vi "ICM Extract Data.vi"(8 "error in (no error)":errorcluster, 11 "Stream File":path) -> (0 "error out":errorcluster, 1 "Stream Data with Separator":string, 2 "Stream Data":string, 3 "Stream File Out":path)   [LabVIEW 2018]
doc: "OSDS Extract Data.vi\n\n This VI opens a Stream file and extracts the data segment.\n\nOCC Streaming Data System Version 1.0\nJune, 2007 Original Code Consulting David Thomson\n www.originalcode.com"
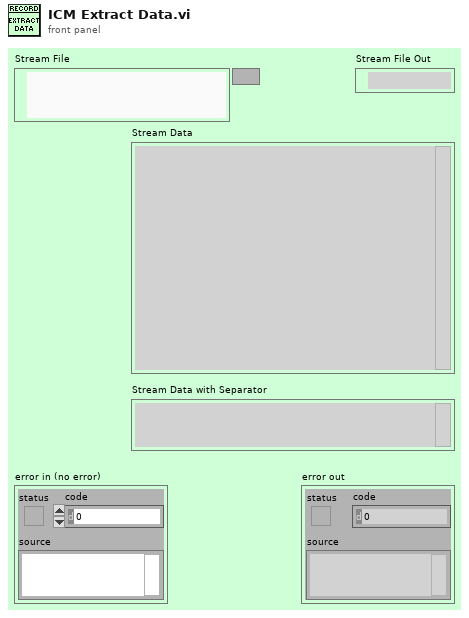
[diagram p1: front panel]
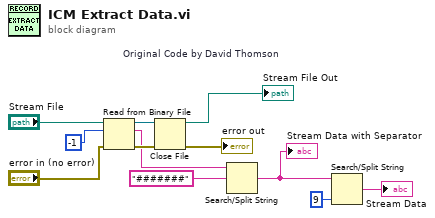
[diagram p0: block diagram]
diagram:
  w12 = "#######"  # Original Code by David Thomson
  n1 = Read from Binary File(8:"error in (no error)", 10:-1 ("count"), 11:"Stream File") -> (0:w6:errorcluster, 2:w4:string, 3:w5:refnum<file>)  [unwired: 3 in, 1 out]
  n2 = Close File(refnum=w5, error in=w6) -> (path=→"Stream File Out":path, error out=→"error out":errorcluster)
  n3 = Search/Split String(string=w4, search string/char (-)=w12) -> (match + rest of string=w10:string)  [unwired: 3 out]
  "Stream Data with Separator" <- w10
  n4 = Search/Split String(string=w10, offset (0)=9) -> (match + rest of string=→"Stream Data":string)  [unwired: 3 out]
